vi "SW_Get_Menu_tags.vi"(0 "Menu ref in":refnum<k9>, 1 "error in (no error)":errorcluster) -> (2 "Menu ref out":refnum<k9>, 3 "(Sub)menu tags":string[](array[string]), 4 "error out":errorcluster)   [LabVIEW 2018, in "Common_Resources.lvlib"]
uses:
  Common_Resources.lvlib
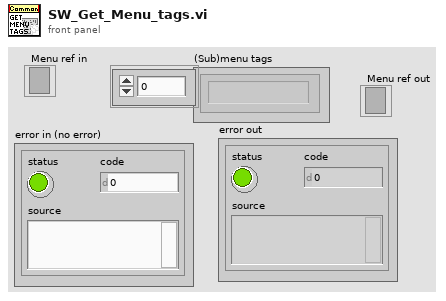
[diagram p1: front panel]
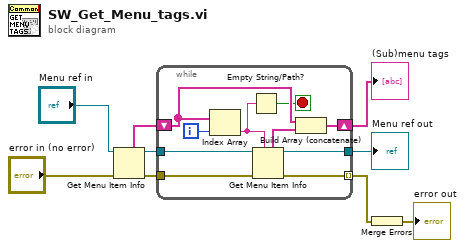
[diagram p0: block diagram]
diagram:
  n1 = Get Menu Item Info(8:"error in (no error)", 11:"Menu ref in") -> (0:w4:errorcluster, 3:w8:refnum<k9>, 5:w7:string[])  [unwired: 1 in, 4 out]
  n2 = while {
    shift-right: [w15] -> w9
    shift-left: w7 -> [w17]
    tunnel: w8 -> [w18]
    tunnel: w4 -> [w12]
    tunnel: [w11] -> w3 mode=indexing
    tunnel: [w10] -> w1
    i -> [w19]
    stop <- w13 stop-if-true
    n3 = Index Array(array=w17, index=w19) -> (element=w14:string)
    n4 = Empty String/Path?(string/path=w14) -> (empty?=w13:bool)
    n5 = Get Menu Item Info(7:w14, 8:w12, 11:w18) -> (0:w11:errorcluster, 3:w10:refnum<k9>, 5:w16:string[])  [unwired: 4 out]
    n6 = Build Array (concatenate)(w17, w16) -> (w15:string[])
  }
  "(Sub)menu tags" <- w9
  "Menu ref out" <- w1
  n7 = Merge Errors(w3) -> (→"error out":errorcluster)
